vi "Read_analog_output.vi"(11 "VISA session":refnum<visa-resource-name>) -> (2 "Still Output":dbl, 3 "Analog Output":dbl)   [LabVIEW 2019]
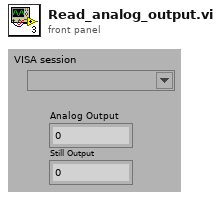
[diagram p1: front panel]
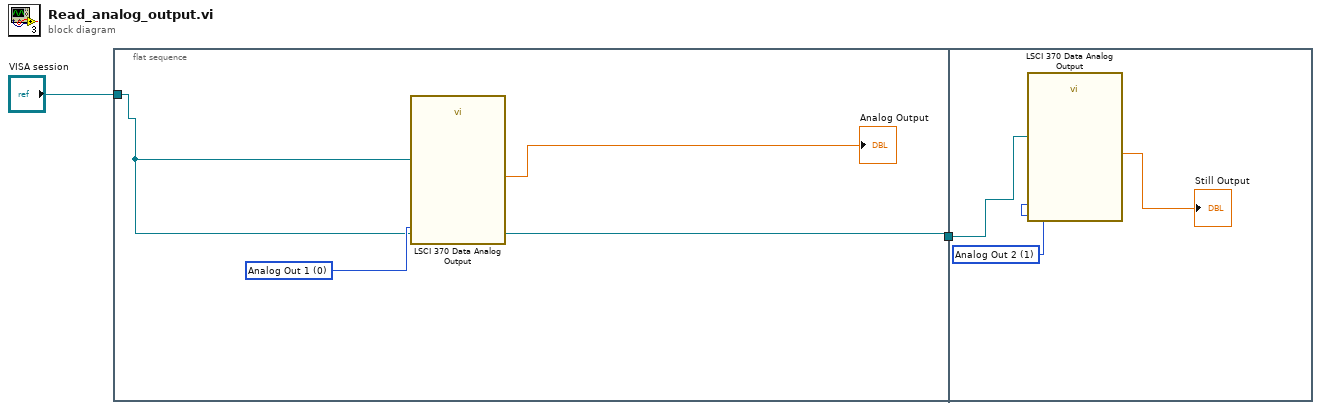
[diagram p0: block diagram]
diagram:
  n1 = flat-sequence {
    tunnel: [w3] -> w2
    tunnel: "VISA session" -> [w3]
    tunnel: w2 -> [w7]
    frame #0 {
      w4 = u16 0 items=["Analog Out 1", "Analog Out 2"] ("Analog Channel (0: Analog Out 1)")
      n2 = call "LSCI 370 Data Analog Output.vi"("VISA session"=w3, "Analog Channel (0: Analog Out 1)"=w4) -> ("Analog Output"=→"Analog Output":dbl)  [unwired: 11 in, 2 out]
    }
    frame #1 {
      w6 = u16 1 items=["Analog Out 1", "Analog Out 2"] ("Analog Channel (0: Analog Out 1)")
      n3 = call "LSCI 370 Data Analog Output.vi"("VISA session"=w7, "Analog Channel (0: Analog Out 1)"=w6) -> ("Analog Output"=→"Still Output":dbl)  [unwired: 11 in, 2 out]
    }
  }
